vi "Dresser DXD Read Pressure (hectoPascal).vi"(0 "VISA session":refnum<visa-resource-name>, 5 "DXD Address (1)":T1=1 min=1 max=99 step=1, 7 "Update Type (Standard)":bool caption="Synchronous\n\nStandard", 11 "Error In (no error)":errorcluster) -> (4 "dup VISA session":refnum<visa-resource-name>, 6 "Returned String":string, 8 "Current Pressure (hectoPascal)":dbl min=-999999.0 max=999999.0 step=1e-05, 10 "Pressure Decimal Position":i32=3 min=0 max=6 step=1, 15 "Error Out":errorcluster)   [LabVIEW 2015]
doc: "This VI will return the current pressure reading, in units of hectoPascal, from the Dresser DXD Series pressure transducer at the specified address. The decimal position of the pressure reading is determined from the value read in.\n\nStandard request for a pressure update will clear the Sr buffer, a pressure update will be performed, and the requested pressure will be shipped out to the interface bus.\n\nThe DXD \"Synchronous Read\" command structure is defined to be a series of two or more commands, depending on the number of DXD units on the RS-485 (RS-232) bus\nThe process begins with the host computer sending the GLOBAL command \"#**Sr\" (This command instructs ALL units on the bus do a pressure conversion and store the result in a buffer (this buffer is called the Sr Buffer). Note that this is a blind command and there is no resonse from any of the units on the bus. The host must then \"time out\" for a predetermined update time determined by the update rate setting of the DXD (13 ms at the fastest update rate of the DXD). After this delay, the Host must query each individual DXD on the bus, by it's unique address, using the proper syntax. This will retrieve the synchronous pressure reading stored in the Sr buffer. After reading the pressure from the Sr buffer, the buffer is cleared. To transmit another reading from the Sr buffer it is necessary for the host to once again start the process by sending another Sr command followed by the previously mentioned timeout, and then request the information from the Sr buffer once again. Requests for information from an empty Sr buffer will result in the generation of a syntax error from the addressed device. It is acceptable to initiate another Sr command sequence is the Sr buffer is currently full. No syntax error will be generated and the new request for a synchronous pressure update will be honored. The new pressure update information will replace that information currently held in the Sr buffer.\n\n\nWritten by:\nBLOOMY CONTROLS, INC\nWINDSOR, CT 06095, USA\n860-298-9925\nwww.bloomy.com\nV2.0.0\nMay, 2002"
uses:
  Type Defs/DXD Address.ctl
panel:
  # "For instructions on the use of this VI, press Ctrl+H to display the help window and move the mouse over the icon, controls, and indicators"
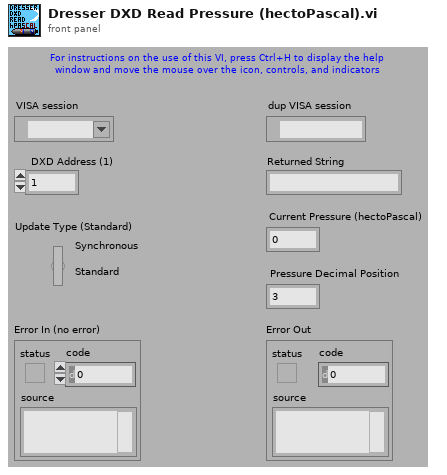
[diagram p1: front panel]
types:
  T1 = typedef "DXD Address.ctl" = i32
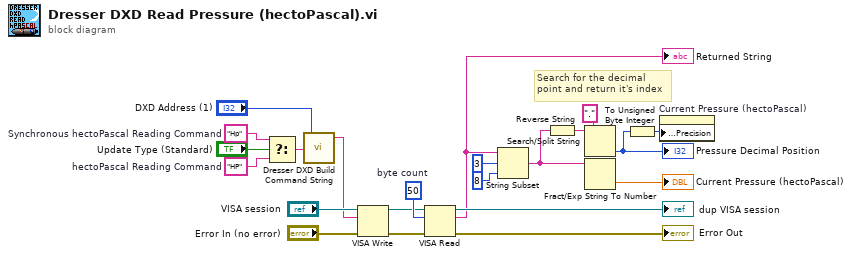
[diagram p0: block diagram]
diagram:
  w4 = "Hp"  # Synchronous hectoPascal Reading Command
  w18 = u32 50  # byte count
  w2 = "HP"  # hectoPascal Reading Command
  # "Search for the decimal\npoint and return it's index"
  n1 = Select(t=w4, s="Update Type (Standard)", f=w2) -> (s? t:f=w1:string)
  n2 = call "Dresser DXD Build Command String.vi"("Command Mnemonic (\"\")"=w1, "DXD Address (1)"="DXD Address (1)") -> ("Command String"=w19:string)  [unwired: 3 in]
  n3 = VISA Write(VISA resource name="VISA session", write buffer=w19, error in (no error)="Error In (no error)") -> (VISA resource name out=w15:refnum<visa-resource-name>, error out=w16:errorcluster)  [unwired: 1 out]
  n4 = VISA Read(VISA resource name=w15, byte count=w18, error in (no error)=w16) -> (VISA resource name out=→"dup VISA session":refnum<visa-resource-name>, read buffer=w5:string, error out=→"Error Out":errorcluster)  [unwired: 1 out]
  "Returned String" <- w5
  n5 = String Subset(string=w5, offset (0)=3, length (rest)=8 ("length (rest)")) -> (substring=w6:string)
  n6 = Reverse String(1:w6) -> (0:w12:string)
  n7 = Search/Split String(string=w12, search string/char (-)="." ("search char (-)")) -> (offset of match=w13:i32)  [unwired: 1 in, 2 out]
  "Pressure Decimal Position" <- w13
  n8 = Fract/Exp String To Number(string=w6) -> (number=→"Current Pressure (hectoPascal)":dbl)  [unwired: 3 in, 1 out]
  n9 = To Unsigned Byte Integer(number=w13) -> (unsigned 8bit integer=w17:u8)
  n10 = property on="Current Pressure (hectoPascal)" class="DigNum (strict)"("Display Format:Precision"=w17) -> ()  [unwired: 2 in, 2 out]
